vi "GoToPosition.vi"(8 "error in (no error)":errorcluster, 10 "Position":dbl[](array[numeric]), 11 "Serial Controller in":refnum<class "Serial Controller.lvclass">) -> (0 "error out":errorcluster, 2 "Moving":bool, 3 "Serial Controller out":refnum<class "Serial Controller.lvclass">)   [LabVIEW 2014, in "Serial Controller.lvclass"]
uses:
  Serial Controller.lvclass
  Serial Controller.lvclass/Serial Controller.ctl
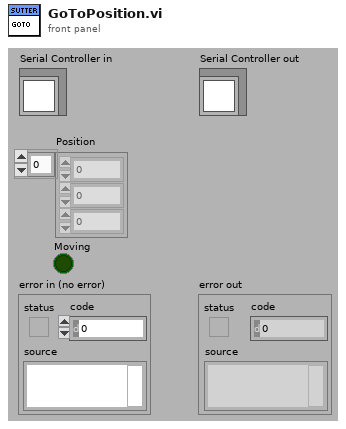
[diagram p1: front panel]
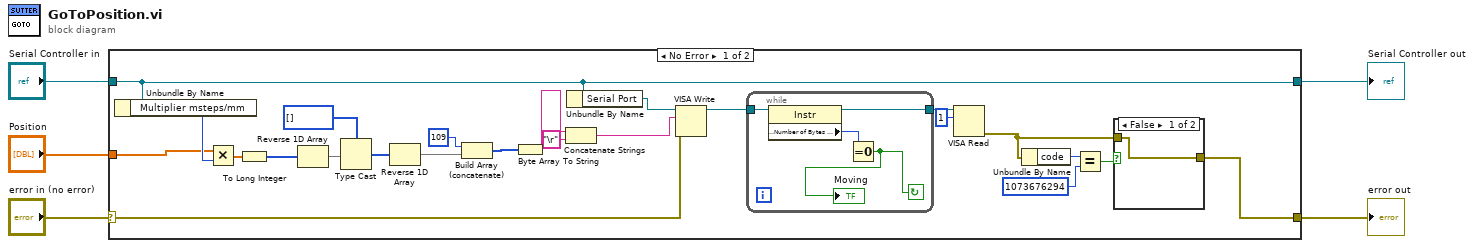
[diagram p0: block diagram]
diagram:
  n1 = case shown="No Error" "error in (no error)" {
    selector: "error in (no error)" -> [w22 w36]
    tunnel: [w16 w36] -> w4
    tunnel: [w23 w35] -> w2
    tunnel: "Serial Controller in" -> [w23 w35]
    tunnel: "Position" -> [w24 _]
    frame No Error {
      n2 = Unbundle By Name(w23) -> ("Multiplier msteps/mm"=w26:i16)
      n3 = Multiply(x=w24, y=w26) -> (x*y=w25:dbl[])
      n4 = To Long Integer(number=w25) -> (32bit integer=w18:i32[])
      n5 = Reverse 1D Array(array=w18) -> (reversed array=w21:i32[])
      n6 = Type Cast(type=u8[] [], x=w21) -> (*(type *) &x=w20:u8[])
      n7 = Reverse 1D Array(array=w20) -> (reversed array=w19:u8[])
      n8 = Build Array (concatenate)(u8 109, w19) -> (w27:u8[])
      n9 = Byte Array To String(unsigned byte array=w27) -> (string=w17:string)
      n10 = Concatenate Strings(w17, "\r" ("string")) -> (w13:string)
      n11 = Unbundle By Name(w23) -> ("Serial Port"=w14:refnum<visa-resource-name>)
      n12 = VISA Write(VISA resource name=w14, write buffer=w13, error in (no error)=w22) -> (VISA resource name out=w12:refnum<visa-resource-name>)  [unwired: 2 out]
      n13 = while {
        tunnel: w12 -> [w34]
        tunnel: [w32] -> w11
        stop <- w31 continue-if-true
        n14 = property class="Instr"(reference=w34) -> (reference out=w32:refnum<visa-resource-name>, "Serial Settings:Number of Bytes at Serial Port"=w33:u32)  [unwired: 1 in, 1 out]
        n15 = Equal To 0?(x=w33) -> (x = 0?=w31:bool)
        "Moving" <- w31
      }
      n16 = VISA Read(VISA resource name=w11, byte count=u32 1) -> (error out=w6:errorcluster)  [unwired: 1 in, 3 out]
      n17 = Unbundle By Name(w6) -> ("code"=w9:i32)
      n18 = Equal?(x=w9, y=1073676294) -> (x = y?=w7:bool)
      n19 = case shown="False" w7 {
        tunnel: w6 -> [w30 _]
        tunnel: [w30 _] -> w16
        frame False {
        }
        frame True {
        }
      }
    }
    frame Error {
    }
  }
  "error out" <- w4
  "Serial Controller out" <- w2
